vi "Trajectory.vi"(6 "Angle(Theta)":dbl, 7 "Height":dbl, 8 "Shooter Height":dbl, 9 "Distance to Hoop (x)":dbl) -> (3 "Velocity":dbl)   [LabVIEW 2011]
panel:
  in  "stop":bool
  in  "Distance from\nSensor to Shooter":dbl
  # "Height of Shooter"
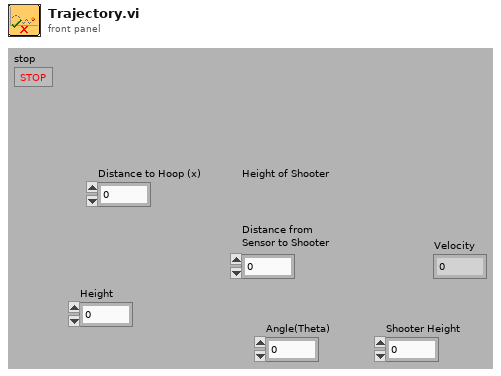
[diagram p1: front panel]
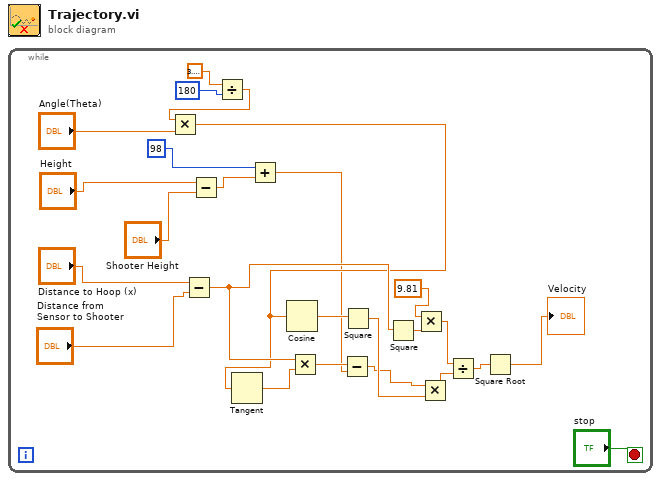
[diagram p0: block diagram]
diagram:
  n1 = while {
    stop <- "stop" stop-if-true
    n2 = Subtract(x="Distance to Hoop (x)", y="Distance from\nSensor to Shooter") -> (x-y=w15:dbl)
    n3 = Subtract(x="Height", y="Shooter Height") -> (x-y=w1:dbl)
    n4 = Divide(x=3.141592653589793, y=180) -> (x/y=w7:dbl)
    n5 = Multiply(x=w7, y="Angle(Theta)") -> (x*y=w6:dbl)
    n6 = Tangent(1:w6) -> (0:w22:dbl)
    n7 = Add(x=98, y=w1) -> (x+y=w4:dbl)
    n8 = Cosine(x=w6) -> (cos(x)=w23:dbl)
    n9 = Multiply(x=w15, y=w22) -> (x*y=w19:dbl)
    n10 = Subtract(x=w19, y=w4) -> (x-y=w16:dbl)
    n11 = Square(x=w23) -> (x^2=w17:dbl)
    n12 = Square(x=w15) -> (x^2=w14:dbl)
    n13 = Multiply(x=9.81, y=w14) -> (x*y=w20:dbl)
    n14 = Multiply(x=w16, y=w17) -> (x*y=w18:dbl)
    n15 = Divide(x=w20, y=w18) -> (x/y=w13:dbl)
    n16 = Square Root(x=w13) -> (sqrt(x)=→"Velocity":dbl)
  }
